vi "SVT Set Swept Sine Distortion Settings.vi"(8 "error in (no error)":errorcluster, 9 "harmonics to visualize":u32[](array[numeric])=[2] min=2, 10 "maximum harmonic":u32=5 min=2, 11 "swept sine task in":T1={"source settings"={"AO task name"="", "source"=[]}, "stimulus settings"={"stimulus task name"="", "stimulus"=[]}, "response(s) settings"={"response task name"="", "response"=[]}, "measurement settings"={"AI sampling frequency"=25600.0, "AO sampling frequency"=25600.0, "AI block size"=2560, "AO block Size"=2560, "block duration [ms]"=100.0, "number of AI channels"=0, "device propagation delay [samples]"=1.0, "total propagation time [samples]"=1.0, "DUT propagation time [ms]"=0.0}, "linlog"=enum."linear", "repeat"=enum."off", "frequency list"=[100.0, 200.0, 300.0, 400.0, 500.0, 600.0, 700.0, 800.0, 900.0, 1000.0, 1100.0, 1200.0, 1300.0, 1400.0, 1500.0, 1600.0, 1700.0, 1800.0, 1900.0, 2000.0, 2100.0, 2200.0, 2300.0, 2400.0, 2500.0, 2600.0, 2700.0, 2800.0, 2900.0, 3000.0, 3100.0, 3200.0, 3300.0, 3400.0, 3500.0, 3600.0, 3700.0, 3800.0, 3900.0, 4000.0, 4100.0, 4200.0, 4300.0, 4400.0, 4500.0, 4600.0, 4700.0, 4800.0, 4900.0, 5000.0, 5100.0, 5200.0, 5300.0, 5400.0, 5500.0, 5600.0, 5700.0, 5800.0, 5900.0, 6000.0, 6100.0, 6200.0, 6300.0, 6400.0, 6500.0, 6600.0, 6700.0, 6800.0, 6900.0, 7000.0, 7100.0, 7200.0, 7300.0, 7400.0, 7500.0, 7600.0, 7700.0, 7800.0, 7900.0, 8000.0, 8100.0, 8200.0, 8300.0, 8400.0, 8500.0, 8600.0, 8700.0, 8800.0, 8900.0, 9000.0, 9100.0, 9200.0, 9300.0, 9400.0, 9500.0, 9600.0, 9700.0, 9800.0, 9900.0, 10000.0], "amplitude list"=[1.414, 1.414, 1.414, 1.414, 1.414, 1.414, 1.414, 1.414, 1.414, 1.414, 1.414, 1.414, 1.414, 1.414, 1.414, 1.414, 1.414, 1.414, 1.414, 1.414, 1.414, 1.414, 1.414, 1.414, 1.414, 1.414, 1.414, 1.414, 1.414, 1.414, 1.414, 1.414, 1.414, 1.414, 1.414, 1.414, 1.414, 1.414, 1.414, 1.414, 1.414, 1.414, 1.414, 1.414, 1.414, 1.414, 1.414, 1.414, 1.414, 1.414, 1.414, 1.414, 1.414, 1.414, 1.414, 1.414, 1.414, 1.414, 1.414, 1.414, 1.414, 1.414, 1.414, 1.414, 1.414, 1.414, 1.414, 1.414, 1.414, 1.414, 1.414, 1.414, 1.414, 1.414, 1.414, 1.414, 1.414, 1.414, 1.414, 1.414, 1.414, 1.414, 1.414, 1.414, 1.414, 1.414, 1.414, 1.414, 1.414, 1.414, 1.414, 1.414, 1.414, 1.414, 1.414, 1.414, 1.414, 1.414, 1.414, 1.414], "settling time"={"settle time"=0.02, "settle cycles"=5}, "integration time"={"integration time"=0.02, "integration cycles"=5}, "frequencies indices"={"AI freq index"=0, "AO freq index"=0}, "read marks"={"write index"=0, "read index"=0, "freq start index"=0, "freq stop index"=0, "# extracted"=0, "buffer type"=enum."Invalid buffer", "read/write indices"=[{"settle time index"=0, "integration time index"=0}, {"settle time index"=0, "integration time index"=0}, {"settle time index"=0, "integration time index"=0}], "AO index"=0, "AI index"=0, "settled"=FALSE, "integration done"=FALSE}, "harmonic settings"={"maximum THD harmonic"=0, "harmonic mapping"=[], "units"={"THD unit"=enum."%", "nth harmonic unit"=enum."%", "SINAD unit"=enum."dB", "THD+N unit"=enum."dB"}}, "auto resolution settings"={"auto max step"=512, "slow threshold db"=6.0, "fast threshold db"=1.0}, "auto level settings"={"auto level enable"=FALSE, "auto level channel"=6, "ideal ref"=1.0, "max level"=10.0, "ref upper deviation db"=3.0, "ref lower deviation db"=-3.0}, "offset"=0.0, "ramping rate"=0.0, "phase"=0.0, "initialize"=FALSE} {"phase" format="%.2f"; "response(s) settings"."response"."channel info"."pregain" format="%.2f"; "response(s) settings"."response"."channel info"."weighting filter" items=["Linear", "A-weighting", "B-weighting", "C-weighting", "ITU-R 468-4", "Dolby", "CCITT", "C-message", "Wb", "Wc", "Wd", "We", "Wf", "Wh", "Wj", "Wk", "Wm", "AES17 20 kHz lowpass", "AES17 40 kHz lowpass", "AES17 20 kHz highpass", "AES17 40 kHz highpass"]; "response(s) settings"."response"."channel info"."dB reference" format="%^.1e"; "response(s) settings"."response"."channel info"."engineering units" items=["custom..."=0, "V"=1, "A"=21, "C"=30, "pC"=31, "s"=32, "-"=29, "Pa"=2, "N"=20, "g"=3, "m/s^2"=4, "m/s"=5, "m"=6, "mm/s"=12, "mm"=13, "micron/s"=14, "micron"=15, "in/s^2"=7, "in/s"=8, "in"=9, "mil/s"=10, "mil"=11, "rad/s^2"=16, "rad/s"=17, "rad"=18, "deg/s^2"=26, "deg/s"=27, "deg"=28, "RPM"=22, "cycle/s^2"=23, "Hz"=24, "cycle"=25, "strain"=19]; "response(s) settings"."response"."channel info"."sensor sensitivity" format="%#_5f"; "stimulus settings"."stimulus"."channel info"."pregain" format="%.2f"; "stimulus settings"."stimulus"."channel info"."weighting filter" items=["Linear", "A-weighting", "B-weighting", "C-weighting", "ITU-R 468-4", "Dolby", "CCITT", "C-message", "Wb", "Wc", "Wd", "We", "Wf", "Wh", "Wj", "Wk", "Wm", "AES17 20 kHz lowpass", "AES17 40 kHz lowpass", "AES17 20 kHz highpass", "AES17 40 kHz highpass"]; "stimulus settings"."stimulus"."channel info"."dB reference" format="%^.1e"; "stimulus settings"."stimulus"."channel info"."engineering units" items=["custom..."=0, "V"=1, "A"=21, "C"=30, "pC"=31, "s"=32, "-"=29, "Pa"=2, "N"=20, "g"=3, "m/s^2"=4, "m/s"=5, "m"=6, "mm/s"=12, "mm"=13, "micron/s"=14, "micron"=15, "in/s^2"=7, "in/s"=8, "in"=9, "mil/s"=10, "mil"=11, "rad/s^2"=16, "rad/s"=17, "rad"=18, "deg/s^2"=26, "deg/s"=27, "deg"=28, "RPM"=22, "cycle/s^2"=23, "Hz"=24, "cycle"=25, "strain"=19]; "stimulus settings"."stimulus"."channel info"."sensor sensitivity" format="%#_5f"; "ramping rate" format="%.4f"; "offset" format="%.2f"; "auto level settings"."ref lower deviation db" format="%.4f"; "auto level settings"."ref upper deviation db" format="%.4f"; "auto level settings"."max level" format="%.4f"; "auto level settings"."ideal ref" format="%.4f"; "auto resolution settings"."fast threshold db" format="%.4f"; "auto resolution settings"."slow threshold db" format="%.4f"; "harmonic settings"."maximum THD harmonic" max=10 step=1; "integration time"."integration time" format="%.2p"; "settling time"."settle time" format="%.2p"; "amplitude list" format="%.2f"; "frequency list" format="%.2f"; "measurement settings"."DUT propagation time [ms]" format="%.2f"; "measurement settings"."AO sampling frequency" format="%.2f"; "measurement settings"."AI sampling frequency" format="%.2f"}) -> (0 "error out":errorcluster={"status"=TRUE, "code"=-1947, "source"="a parameter is invalid"}, 3 "swept sine task out":T1={"source settings"={"AO task name"="", "source"=[]}, "stimulus settings"={"stimulus task name"="", "stimulus"=[]}, "response(s) settings"={"response task name"="", "response"=[]}, "measurement settings"={"AI sampling frequency"=25600.0, "AO sampling frequency"=25600.0, "AI block size"=2560, "AO block Size"=2560, "block duration [ms]"=100.0, "number of AI channels"=0, "device propagation delay [samples]"=1.0, "total propagation time [samples]"=1.0, "DUT propagation time [ms]"=0.0}, "linlog"=enum."linear", "repeat"=enum."off", "frequency list"=[100.0, 200.0, 300.0, 400.0, 500.0, 600.0, 700.0, 800.0, 900.0, 1000.0, 1100.0, 1200.0, 1300.0, 1400.0, 1500.0, 1600.0, 1700.0, 1800.0, 1900.0, 2000.0, 2100.0, 2200.0, 2300.0, 2400.0, 2500.0, 2600.0, 2700.0, 2800.0, 2900.0, 3000.0, 3100.0, 3200.0, 3300.0, 3400.0, 3500.0, 3600.0, 3700.0, 3800.0, 3900.0, 4000.0, 4100.0, 4200.0, 4300.0, 4400.0, 4500.0, 4600.0, 4700.0, 4800.0, 4900.0, 5000.0, 5100.0, 5200.0, 5300.0, 5400.0, 5500.0, 5600.0, 5700.0, 5800.0, 5900.0, 6000.0, 6100.0, 6200.0, 6300.0, 6400.0, 6500.0, 6600.0, 6700.0, 6800.0, 6900.0, 7000.0, 7100.0, 7200.0, 7300.0, 7400.0, 7500.0, 7600.0, 7700.0, 7800.0, 7900.0, 8000.0, 8100.0, 8200.0, 8300.0, 8400.0, 8500.0, 8600.0, 8700.0, 8800.0, 8900.0, 9000.0, 9100.0, 9200.0, 9300.0, 9400.0, 9500.0, 9600.0, 9700.0, 9800.0, 9900.0, 10000.0], "amplitude list"=[1.414, 1.414, 1.414, 1.414, 1.414, 1.414, 1.414, 1.414, 1.414, 1.414, 1.414, 1.414, 1.414, 1.414, 1.414, 1.414, 1.414, 1.414, 1.414, 1.414, 1.414, 1.414, 1.414, 1.414, 1.414, 1.414, 1.414, 1.414, 1.414, 1.414, 1.414, 1.414, 1.414, 1.414, 1.414, 1.414, 1.414, 1.414, 1.414, 1.414, 1.414, 1.414, 1.414, 1.414, 1.414, 1.414, 1.414, 1.414, 1.414, 1.414, 1.414, 1.414, 1.414, 1.414, 1.414, 1.414, 1.414, 1.414, 1.414, 1.414, 1.414, 1.414, 1.414, 1.414, 1.414, 1.414, 1.414, 1.414, 1.414, 1.414, 1.414, 1.414, 1.414, 1.414, 1.414, 1.414, 1.414, 1.414, 1.414, 1.414, 1.414, 1.414, 1.414, 1.414, 1.414, 1.414, 1.414, 1.414, 1.414, 1.414, 1.414, 1.414, 1.414, 1.414, 1.414, 1.414, 1.414, 1.414, 1.414, 1.414], "settling time"={"settle time"=0.02, "settle cycles"=5}, "integration time"={"integration time"=0.02, "integration cycles"=5}, "frequencies indices"={"AI freq index"=0, "AO freq index"=0}, "read marks"={"write index"=0, "read index"=0, "freq start index"=0, "freq stop index"=0, "# extracted"=0, "buffer type"=enum."Invalid buffer", "read/write indices"=[{"settle time index"=0, "integration time index"=0}, {"settle time index"=0, "integration time index"=0}, {"settle time index"=0, "integration time index"=0}], "AO index"=0, "AI index"=0, "settled"=FALSE, "integration done"=FALSE}, "harmonic settings"={"maximum THD harmonic"=0, "harmonic mapping"=[], "units"={"THD unit"=enum."%", "nth harmonic unit"=enum."%", "SINAD unit"=enum."dB", "THD+N unit"=enum."dB"}}, "auto resolution settings"={"auto max step"=512, "slow threshold db"=6.0, "fast threshold db"=1.0}, "auto level settings"={"auto level enable"=FALSE, "auto level channel"=6, "ideal ref"=1.0, "max level"=10.0, "ref upper deviation db"=3.0, "ref lower deviation db"=-3.0}, "offset"=0.0, "ramping rate"=0.0, "phase"=0.0, "initialize"=FALSE} {"phase" format="%.2f"; "response(s) settings"."response"."channel info"."pregain" format="%.2f"; "response(s) settings"."response"."channel info"."weighting filter" items=["Linear", "A-weighting", "B-weighting", "C-weighting", "ITU-R 468-4", "Dolby", "CCITT", "C-message", "Wb", "Wc", "Wd", "We", "Wf", "Wh", "Wj", "Wk", "Wm", "AES17 20 kHz lowpass", "AES17 40 kHz lowpass", "AES17 20 kHz highpass", "AES17 40 kHz highpass"]; "response(s) settings"."response"."channel info"."dB reference" format="%^.1e"; "response(s) settings"."response"."channel info"."engineering units" items=["custom..."=0, "V"=1, "A"=21, "C"=30, "pC"=31, "s"=32, "-"=29, "Pa"=2, "N"=20, "g"=3, "m/s^2"=4, "m/s"=5, "m"=6, "mm/s"=12, "mm"=13, "micron/s"=14, "micron"=15, "in/s^2"=7, "in/s"=8, "in"=9, "mil/s"=10, "mil"=11, "rad/s^2"=16, "rad/s"=17, "rad"=18, "deg/s^2"=26, "deg/s"=27, "deg"=28, "RPM"=22, "cycle/s^2"=23, "Hz"=24, "cycle"=25, "strain"=19]; "response(s) settings"."response"."channel info"."sensor sensitivity" format="%#_5f"; "stimulus settings"."stimulus"."channel info"."pregain" format="%.2f"; "stimulus settings"."stimulus"."channel info"."weighting filter" items=["Linear", "A-weighting", "B-weighting", "C-weighting", "ITU-R 468-4", "Dolby", "CCITT", "C-message", "Wb", "Wc", "Wd", "We", "Wf", "Wh", "Wj", "Wk", "Wm", "AES17 20 kHz lowpass", "AES17 40 kHz lowpass", "AES17 20 kHz highpass", "AES17 40 kHz highpass"]; "stimulus settings"."stimulus"."channel info"."dB reference" format="%^.1e"; "stimulus settings"."stimulus"."channel info"."engineering units" items=["custom..."=0, "V"=1, "A"=21, "C"=30, "pC"=31, "s"=32, "-"=29, "Pa"=2, "N"=20, "g"=3, "m/s^2"=4, "m/s"=5, "m"=6, "mm/s"=12, "mm"=13, "micron/s"=14, "micron"=15, "in/s^2"=7, "in/s"=8, "in"=9, "mil/s"=10, "mil"=11, "rad/s^2"=16, "rad/s"=17, "rad"=18, "deg/s^2"=26, "deg/s"=27, "deg"=28, "RPM"=22, "cycle/s^2"=23, "Hz"=24, "cycle"=25, "strain"=19]; "stimulus settings"."stimulus"."channel info"."sensor sensitivity" format="%#_5f"; "ramping rate" format="%.4f"; "offset" format="%.2f"; "auto level settings"."ref lower deviation db" format="%.4f"; "auto level settings"."ref upper deviation db" format="%.4f"; "auto level settings"."max level" format="%.4f"; "auto level settings"."ideal ref" format="%.4f"; "auto resolution settings"."fast threshold db" format="%.4f"; "auto resolution settings"."slow threshold db" format="%.4f"; "harmonic settings"."maximum THD harmonic" max=10 step=1; "integration time"."integration time" format="%.2p"; "settling time"."settle time" format="%.2p"; "amplitude list" format="%.2f"; "frequency list" format="%.2f"; "measurement settings"."DUT propagation time [ms]" format="%.2f"; "measurement settings"."AO sampling frequency" format="%.2f"; "measurement settings"."AI sampling frequency" format="%.2f"})   [LabVIEW 2017, in "SoundVib_SweptSine.lvlib"]
doc: "Configures the maximum harmonic number and harmonic mapping array used for swept-sine harmonic measurements."
uses:
  <vilib>/addons/Sound and Vibration/svt_Swept Sine/SoundVib_SweptSine.lvlib
  <vilib>/addons/Sound and Vibration/svt_Swept Sine/subVIs/sv_Swept Sine Task.ctl
  <vilib>/addons/_NISVFA/_Shared subVIs/Controls/svc_Channel Info.ctl
  <vilib>/addons/_NISVFA/_Shared subVIs/Controls/svc_Engineering Units Text Ring.ctl
  <vilib>/addons/_NISVFA/_Shared subVIs/Controls/svc_Weighting Filter Text Ring.ctl
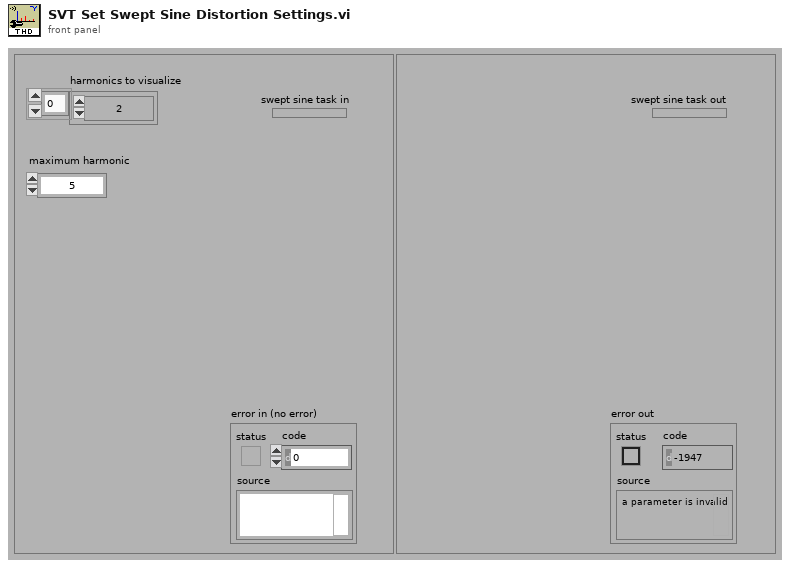
[diagram p1: front panel]
types:
  T1 = typedef "SoundVib_SweptSine.lvlib/sv_Swept Sine Task.ctl" = cluster{"source settings":cluster{"AO task name":refnum<k21>, "source":cluster{"AO physical channel":tag}[]}, "stimulus settings":cluster{"stimulus task name":refnum<k21>, "stimulus":cluster{"stimulus physical channel":tag, "channel info":T2}[]}, "response(s) settings":cluster{"response task name":refnum<k21>, "response":cluster{"response physical channel":tag, "channel info":T2}[]}, "measurement settings":cluster{"AI sampling frequency":dbl, "AO sampling frequency":dbl, "AI block size":i32, "AO block Size":i32, "block duration [ms]":dbl, "number of AI channels":i32, "device propagation delay [samples]":dbl, "total propagation time [samples]":dbl, "DUT propagation time [ms]":dbl}, "linlog":enum16{"linear", "log"}, "repeat":enum16{"off", "on"}, "frequency list":dbl[], "amplitude list":dbl[], "settling time":cluster{"settle time":dbl, "settle cycles":i32}, "integration time":cluster{"integration time":dbl, "integration cycles":i32}, "frequencies indices":cluster{"AI freq index":i32, "AO freq index":i32}, "read marks":cluster{"write index":u32, "read index":u32, "freq start index":u32, "freq stop index":u32, "# extracted":u32, "buffer type":enum16{"Invalid buffer", "Intermediate buffer", "Final buffer"}, "read/write indices":cluster{"settle time index":u32, "integration time index":u32}[], "AO index":i32, "AI index":i32, "settled":bool, "integration done":bool}, "harmonic settings":cluster{"maximum THD harmonic":u32, "harmonic mapping":u32[], "units":cluster{"THD unit":enum16{"dB", "%"}, "nth harmonic unit":enum16{"dB", "%"}, "SINAD unit":enum16{"dB", "%"}, "THD+N unit":enum16{"dB", "%"}}}, "auto resolution settings":cluster{"auto max step":i32, "slow threshold db":dbl, "fast threshold db":dbl}, "auto level settings":cluster{"auto level enable":bool, "auto level channel":u8, "ideal ref":sgl, "max level":sgl, "ref upper deviation db":sgl, "ref lower deviation db":sgl}, "offset":dbl, "ramping rate":dbl, "phase":dbl, "initialize":bool}
  T2 = typedef "svc_Channel Info.ctl" = cluster{"sensor sensitivity":dbl, "engineering units":T3, "dB reference":dbl, "custom label":string, "weighting filter":T4, "pregain":dbl}
  T3 = typedef "svc_Engineering Units Text Ring.ctl" = u16
  T4 = typedef "svc_Weighting Filter Text Ring.ctl" = u16
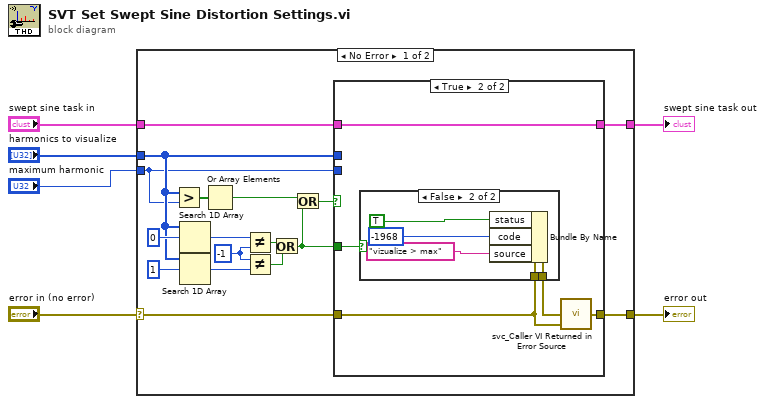
[diagram p0: block diagram]
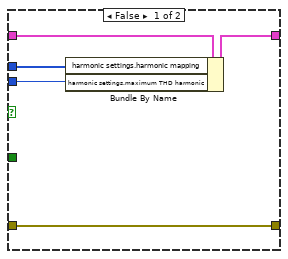
[diagram p2: hidden frame]
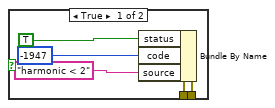
[diagram p3: hidden frame]
diagram:
  n1 = case shown="No Error" "error in (no error)" {
    selector: "error in (no error)" -> [w13 w44]
    tunnel: "swept sine task in" -> [w11 w45]
    tunnel: [w10 w45] -> w5
    tunnel: "maximum harmonic" -> [w8 _]
    tunnel: "harmonics to visualize" -> [w9 _]
    tunnel: [w12 w44] -> w1
    frame No Error {
      w18 = -1 ("y")
      n2 = Greater?(x=w9, y=w8) -> (0:w23:bool[])
      n3 = Search 1D Array(1D array=w9, element=u32 0) -> (index of element=w20:i32)  [unwired: 1 in]
      n4 = Search 1D Array(1D array=w9, element=u32 1) -> (index of element=w19:i32)  [unwired: 1 in]
      n5 = Or Array Elements(Boolean array=w23) -> (logical OR=w15:bool)
      n6 = Not Equal?(x=w20, y=w18) -> (x != y?=w17:bool)
      n7 = Not Equal?(x=w18, y=w19) -> (x != y?=w16:bool)
      n8 = Or(x=w17, y=w16) -> (x .or. y?=w7:bool)
      n9 = Or(x=w15, y=w7) -> (x .or. y?=w14:bool)
      n10 = case shown="True" w14 {
        tunnel: w13 -> [w28 w29]
        tunnel: [w28 w32] -> w12
        tunnel: w11 -> [w25 w33]
        tunnel: [w24 w33] -> w10
        tunnel: w9 -> [w27 _]
        tunnel: w8 -> [w26 _]
        tunnel: w7 -> [_ w30]
        frame False {
          n11 = Bundle By Name(cluster=w25, "harmonic settings.harmonic mapping"=w27, "harmonic settings.maximum THD harmonic"=w26) -> (w24:T1)
        }
        frame True {
          n12 = case shown="False" w30 {
            tunnel: w29 -> [w38 w43]
            tunnel: [w37 w42] -> w31
            frame True {
              n13 = Bundle By Name(cluster=w38, "status"=TRUE, "code"=-1947, "source"="harmonic < 2") -> (w37:errorcluster)
            }
            frame False {
              n14 = Bundle By Name(cluster=w43, "status"=TRUE, "code"=-1968, "source"="vizualize > max") -> (w42:errorcluster)
            }
          }
          n15 = call <vilib>:"svc_Caller VI Returned in Error Source.vi"("warning input to caller"=w29, "error in (no error)"=w31) -> ("error out"=w32:errorcluster)  [unwired: 3 in]
        }
      }
    }
    frame Error {
    }
  }
  "error out" <- w1
  "swept sine task out" <- w5
